vi "Programmsequenz.vi"(8 "Programm":T1[](array[typedef]), 9 "Prozessvariable Nr. N":i32, 10 "Stellung x (0..9)":i16, 11 "Zuordnungtabelle":i16[][](array[numeric])) -> (0 "Sequenz":T1[](array[typedef]), 5 "Länge":i16)   [LabVIEW 2020, in "Anlagenuebersicht.lvlib" / "VisBx Anzeige.lvlib"]
doc: "Holt mit Hilfe der Zuordnungstabelle aus dem Programm für den Aufbau eines Bewegtbildes jene Sequenz von Zeichenbefehlen (mit Parametern), die zur Darstellung der Prozessvariablen Nr. N in der aktuellen Stellung x gebraucht werden.\n\nZuordnungstabelle:\nSpalte 0: voriges x bzw. Palette\nSpalte 1: steuerndes N\nSpalte 2: Nachkommastellen\nSpalte 3: Stellungstyp\n\nSpalte 4: Programmindex für x=0\nSpalte 5: Anzahl der Programm-Schritte für x=0\n\nSpalte 6: Programmindex für x=1\nSpalte 7: Anzahl der Programm-Schritte für x=1\n....\n....\nSpalte 22: Programmindex für x=9\nSpalte 23: Anzahl der Programm-Schritte für x=9"
uses:
  VisBx Anzeige.lvlib
  VisParameter/VisSchritt.ctl
  VisParameter/VisSchritt-Typ.ctl
  VisParameter/VisParam-Typdef.lvlib
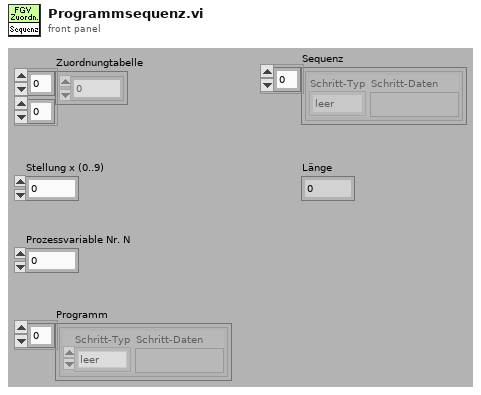
[diagram p1: front panel]
types:
  T1 = typedef "VisParam-Typdef.lvlib/VisSchritt.ctl" = cluster{"Schritt-Typ":T2, "Schritt-Daten":variant}
  T2 = typedef "VisParam-Typdef.lvlib/VisSchritt-Typ.ctl" = enum16{"leer", "Punkt", "Linie", "Linienzug", "Fixtext", "Textrechteck", "Ziffernanzeige", "Rechteck", "Rechteck rund", "Ellipse", "Bogen", "Kreis", "Pixmap"}
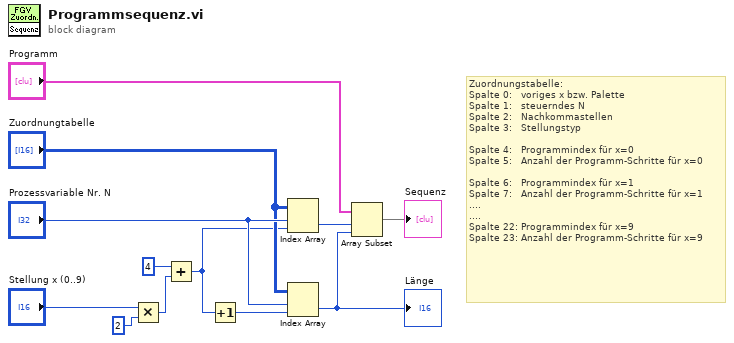
[diagram p0: block diagram]
diagram:
  # "Zuordnungstabelle:\nSpalte 0:   voriges x bzw. Palette\nSpalte 1:   steuerndes N\nSpalte 2:   Nachkommastellen\nSpalte 3:   Stellungstyp\n\nSpalte 4:   Programmindex für x=0\nSpalte 5:   Anzahl der Programm-Schritte für x=0\n\nSpalte 6:   Programmindex für x=1\nSpalte 7:   Anzahl der Programm-Schritte für x=1\n....\n....\nSpalte 22: Programmindex für x=9\nSpalte 23: Anzahl der Programm-Schritte für x=9"
  n1 = Multiply(x="Stellung x (0..9)", y=u16 2) -> (x*y=w3:u16)
  n2 = Add(x=u16 4, y=w3) -> (x+y=w1:u16)
  n3 = Increment(x=w1) -> (x+1=w6:u16)
  n4 = Index Array ("Array indizieren")(array="Zuordnungtabelle", index (row)="Prozessvariable Nr. N", index (col)=w1) -> (element=w9:i16)
  n5 = Index Array ("Array indizieren")(array="Zuordnungtabelle", index (row)="Prozessvariable Nr. N", index (col)=w6) -> (element=w10:i16)
  "Länge" <- w10
  n6 = Array Subset(array="Programm", index=w9, length=w10) -> (→"Sequenz":T1[])
